vi "Check and Override Channel Configuration.vi"(8 "error in (no error)":errorcluster, 10 "Custom Config Data in":u8[](array[numeric]) format="%.0x", 11 "CIFChannels in":refnum<class "CIF_NIChn_Fifo_Power.lvclass">) -> (0 "error out":errorcluster, 2 "Custom Config Data out":u8[](array[numeric]) format="%.0x", 3 "CIFChannels out":refnum<class "CIF_NIChn_Fifo_Power.lvclass">)   [LabVIEW 2021, in "CIF_NIChn_Fifo_Power.lvclass"]
uses:
  CIF_NIChn_Fifo_Power.lvclass
  <vilib>/CIF Foundation/CIF Utilities/DataTypes/Unflatten U64.vi
  <vilib>/CIF Foundation/CIF Utilities/DataTypes/Flatten U64.vi
  ChannelCommon/ChannelCommon.lvlib
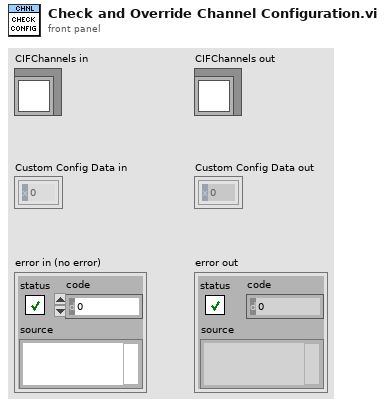
[diagram p1: front panel]
types:
  T1 = typedef "ChannelCommon.lvlib/FIFO Config.ctl" = cluster{"Max Bytes/Msg":u64, "Max Msg/FIFO":u64, "Flags":u64}
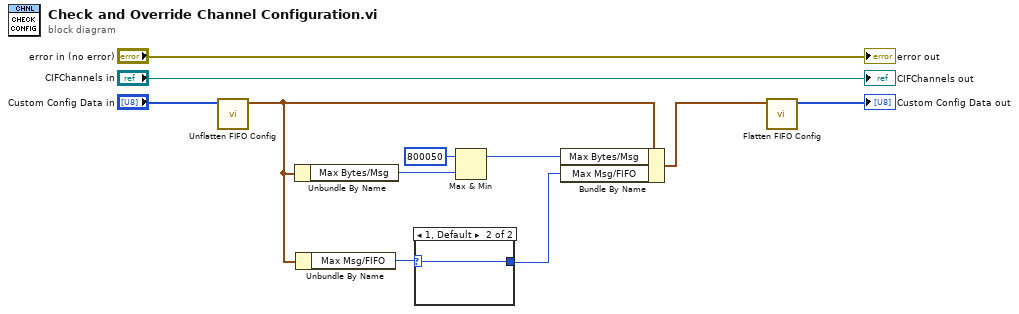
[diagram p0: block diagram]
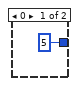
[diagram p2: hidden frame]
diagram:
  n1 = call "Unflatten FIFO Config.vi"("Flattened Data in"="Custom Config Data in") -> ("FIFO Config out"=w7:T1)  [unwired: 9 in, 1 out]
  n2 = Unbundle By Name(w7) -> ("Max Bytes/Msg"=w4:u64)
  n3 = Unbundle By Name(w7) -> ("Max Msg/FIFO"=w6:u64)
  n4 = case shown="1, Default" w6 {
    selector: w6 -> [_ w13]
    tunnel: [u64 5 ("Max Msg/FIFO") w13] -> w5
    frame 0 {
    }
    frame 1, Default {
    }
  }
  n5 = Max & Min(x=u64 800050, y=w4) -> (max(x,y)=w3:u64)  [unwired: 1 out]
  n6 = Bundle By Name(cluster=w7, "Max Bytes/Msg"=w3, "Max Msg/FIFO"=w5) -> (w8:T1)
  n7 = call "Flatten FIFO Config.vi"("FIFO Config in"=w8) -> ("Flattened FIFO Config"=→"Custom Config Data out":u8[])  [unwired: 10 in]
  "CIFChannels out" <- "CIFChannels in"
  "error out" <- "error in (no error)"
